vi "SS Class Init.vi"(7 "VI Refnum":refnum<vi>, 8 "error in (no error)":errorcluster, 9 "Init Data":variant, 10 "Device":string, 11 "Subsystem Class in":refnum<class "Subsystem Class.lvclass">) -> (0 "error out":errorcluster, 2 "Channel List":refnum<class "HK Item.lvclass">[](array[class]), 3 "Subsystem Class out":refnum<class "Subsystem Class.lvclass">)   [LabVIEW 2021, in "Subsystem Class.lvclass"]
uses:
  Subsystem Class.lvclass
  hk-channel-class/HK Item/HK Item.lvclass
  SS typedef cluster Instrument Command Queue Data.ctl
  Subsystem Class.lvclass/Subsystem Class.ctl
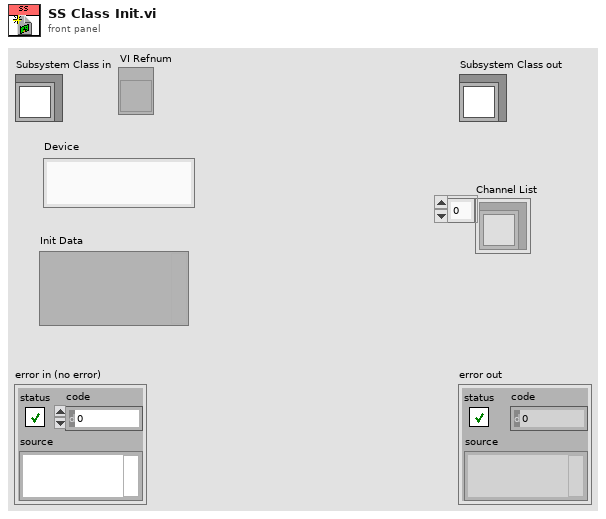
[diagram p1: front panel]
types:
  T1 = typedef "SS typedef cluster Instrument Command Queue Data.ctl" = cluster{"Cmd":string, "Parameters":variant}
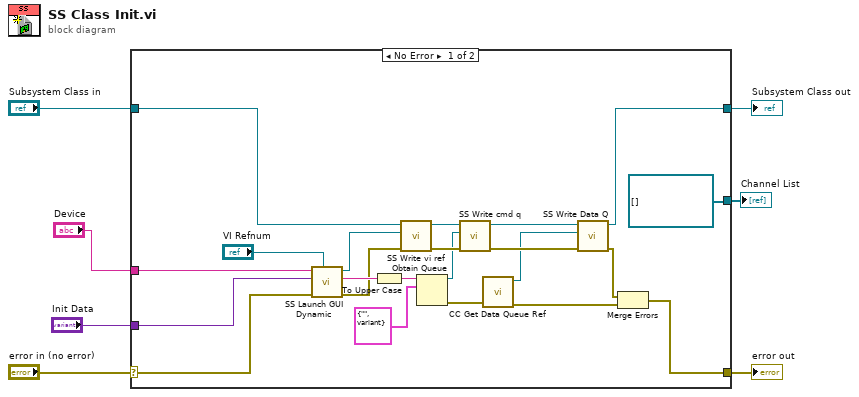
[diagram p0: block diagram]
diagram:
  n1 = case shown="No Error" "error in (no error)" {
    selector: "error in (no error)" -> [w16 w31]
    tunnel: [w13 w31] -> w6
    tunnel: [w10 w30] -> w4
    tunnel: "Subsystem Class in" -> [w12 w30]
    tunnel: "Device" -> [w18 _]
    tunnel: "Init Data" -> [w17 _]
    tunnel: [refnum<class "HK Item.lvclass">[] [] ("Channel List") _] -> w1
    frame No Error {
      n2 = call "SS Launch GUI Dynamic.vi"("VI Refnum"="VI Refnum", "error in (no error)"=w16, "Data"=w17, "Device Name"=w18) -> ("error out"=w26:errorcluster, "VI Clone Name"=w27:string, "reference out"=w8:refnum<vi>)  [unwired: 5 in]
      n3 = To Upper Case(1:w27) -> (0:w28:string)
      n4 = call "SS Write vi ref.vi"("error in (no error)"=w26, "reference out"=w8, "Subsystem Class in"=w12) -> ("error out"=w25:errorcluster, "Subsystem Class out"=w24:refnum<class "Subsystem Class.lvclass">)  [unwired: 7 in]
      n5 = Obtain Queue(name (unnamed)=w28, element data type=T1 {"Cmd"="", "Parameters"=variant}) -> (queue out=w23:refnum<queue>, error out=w21:errorcluster)  [unwired: 3 in, 1 out]
      n6 = call "SS Write cmd q.vi"("error in (no error)"=w25, "cmd q"=w23, "Subsystem Class in"=w24) -> ("error out"=w22:errorcluster, "Subsystem Class out"=w20:refnum<class "Subsystem Class.lvclass">)  [unwired: 7 in]
      n7 = call "CC Get Data Queue Ref.vi"("error in (no error)"=w21) -> ("error out"=w15:errorcluster, "Data Q"=w19:refnum<queue>)  [unwired: 9 in]
      n8 = call "SS Write Data Q.vi"("error in (no error)"=w22, "Data Q"=w19, "Subsystem Class in"=w20) -> ("error out"=w14:errorcluster, "Subsystem Class out"=w10:refnum<class "Subsystem Class.lvclass">)  [unwired: 7 in]
      n9 = Merge Errors(w14, w15) -> (w13:errorcluster)
    }
    frame Error {
    }
  }
  "error out" <- w6
  "Subsystem Class out" <- w4
  "Channel List" <- w1
